vi "Seconds to Time.vi"(10 "Seconds":i32) -> (2 "Time String":string)   [LabVIEW 2020, in "hse-misc.lvlib"]
doc: "Convert a time range (in seconds) to a time string in the format \"hh:mm:ss\".\nE.g. 3680s -> \"01:01:20\".\n\n____\nHAMPEL SOFTWARE ENGINEERING v3.8.0 (2023-12-18 14:41)"
uses:
  hse-misc.lvlib
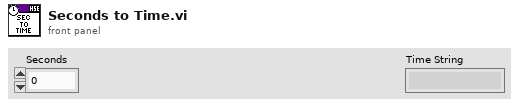
[diagram p1: front panel]
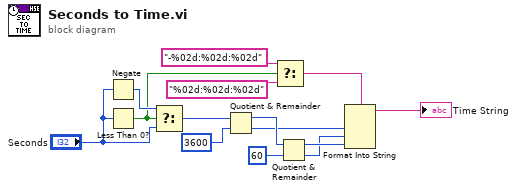
[diagram p0: block diagram]
diagram:
  n1 = Negate(x="Seconds") -> (-x=w7:i32)
  n2 = Less Than 0?(x="Seconds") -> (x < 0?=w4:bool)
  n3 = Select(t=w7, s=w4, f="Seconds") -> (s? t:f=w5:i32)
  n4 = Quotient & Remainder(x=w5, y=3600) -> (x-y*floor(x/y)=w13:i32, floor(x/y)=w12:i32)
  n5 = Select(t="-%02d:%02d:%02d" ("format string"), s=w4, f="%02d:%02d:%02d" ("format string")) -> (s? t:f=w2:string)
  n6 = Quotient & Remainder(x=w13, y=60) -> (x-y*floor(x/y)=w10:i32, floor(x/y)=w9:i32)
  n7 = Format Into String(format string=w2, w12, w9, w10) -> (resulting string=→"Time String":string)  [unwired: 2 in, 1 out]
